vi "Waveform Generator.vi"() -> ()   [LabVIEW 2015]
panel:
  out "XY Graph":cluster{"X":dbl, "Y":dbl}[](graph)
  in  "Stop":bool
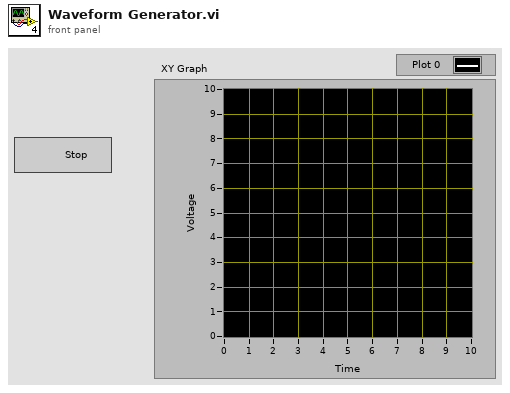
[diagram p1: front panel]
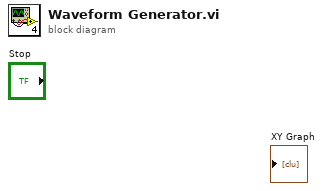
[diagram p0: block diagram]
diagram:
